vi "IsInput.vi"(6 "error in":errorcluster, 9 "Tunnel in":refnum<class "FlatSequenceInnerTunnel.lvclass">) -> (0 "error out":errorcluster, 3 "Tunnel out":refnum<class "FlatSequenceInnerTunnel.lvclass">, 4 "Input":bool)   [LabVIEW 2014, in "FlatSequenceInnerTunnel.lvclass"]
uses:
  FlatSequenceInnerTunnel.lvclass
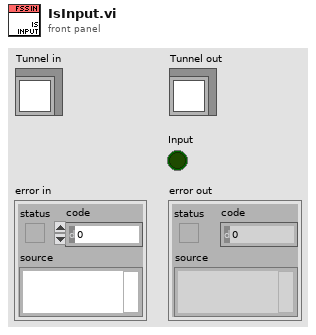
[diagram p1: front panel]
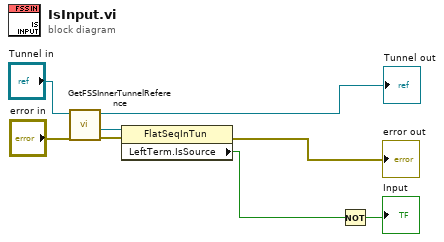
[diagram p0: block diagram]
diagram:
  n1 = call "GetFSSInnerTunnelReference.vi"("error in"="error in", "Tunnel in"="Tunnel in") -> ("error out"=w6:errorcluster, "reference out"=w5:refnum<vi>, "Tunnel out"=→"Tunnel out":refnum<class "FlatSequenceInnerTunnel.lvclass">)  [unwired: 7 in]
  n2 = property class="FlatSeqInTun"(reference=w5, error in=w6) -> (error out=→"error out":errorcluster, "LeftTerm.IsSource"=w2:bool)  [unwired: 1 out]
  n3 = Not(x=w2) -> (.not. x?=→"Input":bool)
